vi "VI Tree.vi"   [LabVIEW 2023, in "Stanford Research 830.lvlib"]
doc: "This is the instrument driver for the Stanford Research 810/830. The VI Tree displays all the user-callable VIs of the instrument driver in an organized table."
uses:
  Stanford Research 830.lvlib
  Data/Read (Multiple Points).vi
  Data/Read (All Parameters).vi
  Data/Read (1 Parameter).vi
panel:
  # "(c) 2006 National Instruments.  ALL RIGHTS RESERVED."
  # "SEE DIAGRAM\nFOR VI TREE."
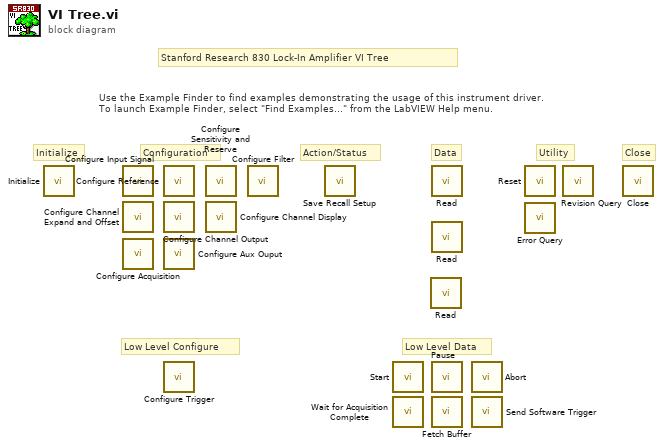
[diagram p0: block diagram]
diagram:
  # "Low Level Configure"
  # "Close"
  # "Utility"
  # "Data"
  # "Action/Status"
  # "Configuration"
  # "Initialize"
  # "Low Level Data"
  # "Stanford Research 830 Lock-In Amplifier VI Tree"
  # "Use the Example Finder to find examples demonstrating the usage of this instrument driver.\nTo launch Example Finder, select \"Find Examples...\" from the LabVIEW Help menu."
  n1 = call "Initialize.vi"() -> ()  [unwired: 10 in, 2 out]
  n2 = call "Configure Input Signal.vi"() -> ()  [unwired: 10 in, 2 out]
  n3 = call "Configure Channel Expand and Offset.vi"() -> ()  [unwired: 10 in, 2 out]
  n4 = call "Configure Acquisition.vi"() -> ()  [unwired: 10 in, 2 out]
  n5 = call "Configure Reference.vi"() -> ()  [unwired: 14 in, 2 out]
  n6 = call "Configure Channel Output.vi"() -> ()  [unwired: 10 in, 2 out]
  n7 = call "Configure Aux Ouput.vi"() -> ()  [unwired: 10 in, 2 out]
  n8 = call "Configure Trigger.vi"() -> ()  [unwired: 10 in, 2 out]
  n9 = call "Configure Sensitivity and Reserve.vi"() -> ()  [unwired: 10 in, 2 out]
  n10 = call "Configure Channel Display.vi"() -> ()  [unwired: 10 in, 2 out]
  n11 = call "Configure Filter.vi"() -> ()  [unwired: 10 in, 2 out]
  n12 = call "Save Recall Setup.vi"() -> ()  [unwired: 10 in, 2 out]
  n13 = call "Start.vi"() -> ()  [unwired: 10 in, 2 out]
  n14 = call "Wait for Acquisition Complete.vi"() -> ()  [unwired: 10 in, 2 out]
  n15 = call-poly "Read.vi"() -> ()  [unwired: 9 in, 3 out]
  n16 = call-poly "Read.vi"() -> ()  [unwired: 9 in, 3 out]
  n17 = call-poly "Read.vi"() -> ()  [unwired: 9 in, 3 out]
  n18 = call "Pause.vi"() -> ()  [unwired: 10 in, 2 out]
  n19 = call "Fetch Buffer.vi"() -> ()  [unwired: 9 in, 3 out]
  n20 = call "Abort.vi"() -> ()  [unwired: 10 in, 2 out]
  n21 = call "Send Software Trigger.vi"() -> ()  [unwired: 10 in, 2 out]
  n22 = call "Reset.vi"() -> ()  [unwired: 10 in, 2 out]
  n23 = call "Error Query.vi"() -> ()  [unwired: 9 in, 3 out]
  n24 = call "Revision Query.vi"() -> ()  [unwired: 8 in, 4 out]
  n25 = call "Close.vi"() -> ()  [unwired: 11 in, 1 out]
